vi "ActionVIOnSave (File).vi"(8 "error in":errorcluster, 11 "file item reference in":T1 format="%.0x") -> (0 "error out":errorcluster, 3 "file item reference out":T1 format="%.0x")   [LabVIEW 2027, in "Embedded Data Logger System Explorer.lvlib"]
uses:
  Embedded Data Logger System Explorer.lvlib
  <vilib>/NI VeriStand/Custom Device API/Custom Device Item Ref.ctl
  Scripting/Embedded Data Logger Scripting.lvlib
  <vilib>/NI VeriStand/Custom Device API/Custom Device API.lvlib
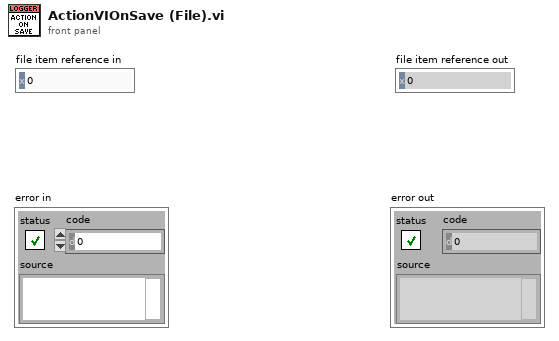
[diagram p1: front panel]
types:
  T1 = typedef "Custom Device API.lvlib/Custom Device Item Ref.ctl" = u64
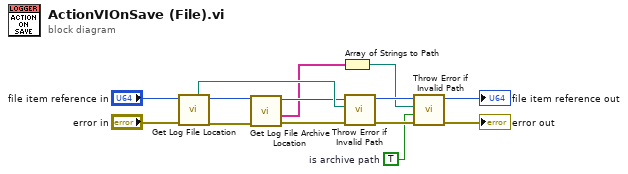
[diagram p0: block diagram]
diagram:
  w12 = TRUE  # is archive path
  n1 = call "Get Log File Location.vi"("error in (no error)"="error in", "log file in"="file item reference in") -> ("error out"=w3:errorcluster, "log file out"=w6:T1, "sample path"=w7:path)  [unwired: 4 in, 3 out]
  n2 = call "Get Log File Archive Location.vi"("error in (no error)"=w3, "log file in"=w6) -> ("error out"=w4:errorcluster, "archive directory parts"=w2:string[], "log file out"=w5:T1)  [unwired: 6 in, 1 out]
  n3 = Array of Strings to Path(0:w2) -> (2:w1:path)  [unwired: 1 in]
  n4 = call "Throw Error if Invalid Path.vi"("error in"=w4, "file path"=w7, "item reference in"=w5) -> ("error out"=w14:errorcluster, "item reference out"=w13:T1)  [unwired: 7 in]
  n5 = call "Throw Error if Invalid Path.vi"("error in"=w14, "is archive path"=w12, "file path"=w1, "item reference in"=w13) -> ("error out"=→"error out":errorcluster, "item reference out"=→"file item reference out":T1)  [unwired: 6 in]
